vi "Set Master Scan Enable.vi"(8 "error in (no error)":errorcluster, 10 "Set Master Scan Enable?":bool, 11 "hdl in":i32) -> (0 "error out":errorcluster, 3 "hdl":i32)   [LabVIEW 2011, in "Thorlabs_MDT69xB.lvlib"]
doc: "Sets Master Scan mode."
uses:
  <instrlib>/Thorlabs_MDT69xB/Thorlabs_MDT69xB.lvlib
  <instrlib>/Thorlabs_MDT69xB/Data/MDT_COMMAND_LIB_win32.dll
  <instrlib>/Thorlabs_MDT69xB/Data/MDT_COMMAND_LIB_x64.dll
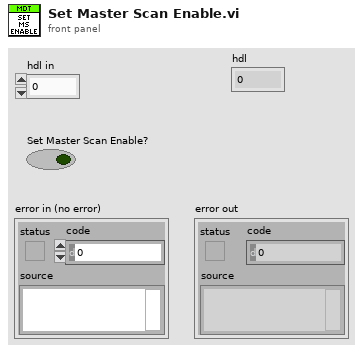
[diagram p1: front panel]
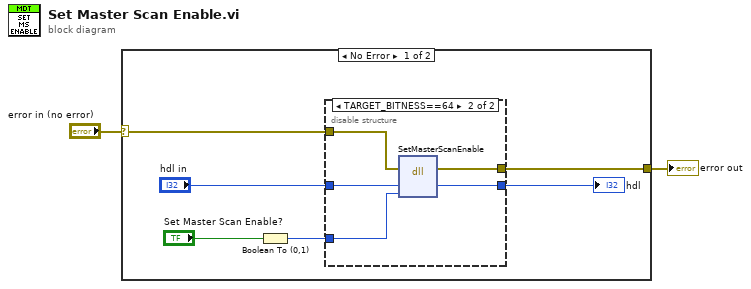
[diagram p0: block diagram]
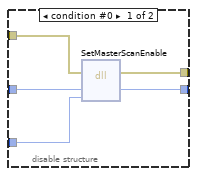
[diagram p2: hidden frame]
diagram:
  n1 = case shown="No Error" "error in (no error)" {
    selector: "error in (no error)" -> [w5 w19]
    tunnel: [w4 w19] -> w1
    frame No Error {
      n2 = Boolean To (0,1)(Boolean="Set Master Scan Enable?") -> (0, 1=w7:i16)
      n3 = disable-structure shown="TARGET_BITNESS==64" {
        disable-tunnel: w7 -> [w13 w18]
        disable-tunnel: "hdl in" -> [w12 w17]
        disable-tunnel: w5 -> [w11 w16]
        disable-tunnel: [w10 w15] -> w4
        disable-tunnel: [w9 w14] -> w3
        frame condition #0 {
          n4 = dll-call lib="E:/Program Files (x86)/National Instruments/LabVIEW 2011/instr.lib/Thorlabs_MDT69xB/Data/MDT_COMMAND_LIB_win32.dll" fn="SetMasterScanEnable"(error in=w11, "hdl"=w12, "state"=w13) -> (error out=w10:errorcluster, "hdl"=w9:i32)  [unwired: 4 in, 1 out]
        }
        frame condition #1 (active) {
          n5 = dll-call lib="C:/Program Files/National Instruments/LabVIEW 2011/instr.lib/Thorlabs_MDT69xB/Data/MDT_COMMAND_LIB_x64.dll" fn="SetMasterScanEnable"(error in=w16, "hdl"=w17, "state"=w18) -> (error out=w15:errorcluster, "hdl"=w14:i32)  [unwired: 4 in, 1 out]
        }
      }
      "hdl" <- w3
    }
    frame Error {
    }
  }
  "error out" <- w1
